vi "RW RxTx.vi"(8 "error in (no error)":errorcluster) -> (0 "error out":errorcluster)   [LabVIEW 2018]
uses:
  RxTx/CCS_RxTx.lvclass
  <vilib>/addons/_JKI Toolkits/Caraya/classes/Assert/Assert Equal Value_Variant.vi
  <vilib>/addons/_JKI Toolkits/Caraya/classes/Test/Test.lvclass
  <vilib>/addons/_JKI Toolkits/Caraya/classes/Assert/Assert.lvclass
panel:
  in  "RxTx in":refnum<class "CCS_RxTx.lvclass">
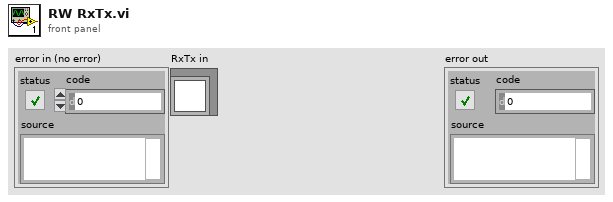
[diagram p1: front panel]
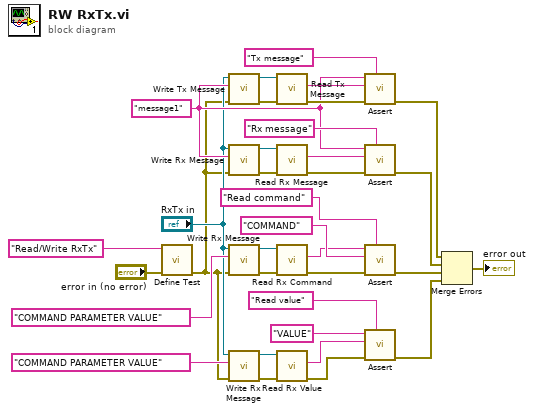
[diagram p0: block diagram]
diagram:
  w19 = "message1" ("Label (VI Title)")
  n1 = call <vilib>:"Define Test.vi"("error in (no error)"="error in (no error)", "Label (VI Title)"="Read/Write RxTx") -> ("error out"=w2:errorcluster)  [unwired: 8 in, 1 out]
  n2 = call "Write Tx Message.vi"("error in (no error)"=w2, "Tx Message"=w19, "RxTx in"="RxTx in") -> ("error out"=w31:errorcluster, "RxTx out"=w23:refnum<class "CCS_RxTx.lvclass">)  [unwired: 7 in]
  n3 = call "Write Rx Message.vi"("error in (no error)"=w2, "Rx Message"=w19, "RxTx in"="RxTx in") -> ("error out"=w28:errorcluster, "RxTx out"=w22:refnum<class "CCS_RxTx.lvclass">)  [unwired: 7 in]
  n4 = call "Write Rx Message.vi"("error in (no error)"=w2, "Rx Message"="COMMAND PARAMETER VALUE" ("Label (VI Title)"), "RxTx in"="RxTx in") -> ("error out"=w16:errorcluster, "RxTx out"=w15:refnum<class "CCS_RxTx.lvclass">)  [unwired: 7 in]
  n5 = call "Write Rx Message.vi"("error in (no error)"=w2, "Rx Message"="COMMAND PARAMETER VALUE" ("Label (VI Title)"), "RxTx in"="RxTx in") -> ("error out"=w9:errorcluster, "RxTx out"=w8:refnum<class "CCS_RxTx.lvclass">)  [unwired: 7 in]
  n6 = call "Read Tx Message.vi"("error in (no error)"=w31, "RxTx in"=w23) -> ("error out"=w30:errorcluster, "Tx Message"=w20:string)  [unwired: 7 in, 1 out]
  n7 = call "Read Rx Message.vi"("error in (no error)"=w28, "RxTx in"=w22) -> ("error out"=w27:errorcluster, "Rx Message"=w21:string)  [unwired: 7 in, 1 out]
  n8 = call "Read Rx Command.vi"("error in (no error)"=w16, "RxTx in"=w15) -> ("error out"=w17:errorcluster, "Rx Command"=w12:string)  [unwired: 7 in, 1 out]
  n9 = call "Read Rx Value.vi"("error in (no error)"=w9, "RxTx in"=w8) -> ("error out"=w1:errorcluster, "Rx value"=w7:string)  [unwired: 7 in, 1 out]
  n10 = call-poly <vilib>:"Assert.vi"("Label"="Tx message" ("Label (VI Title)"), "error in (no error)"=w30, "Y"=w20, "X"=w19) -> ("error out"=w32:errorcluster)  [unwired: 6 in, 1 out]
  n11 = call-poly <vilib>:"Assert.vi"("Label"="Rx message" ("Label (VI Title)"), "error in (no error)"=w27, "Y"=w21, "X"=w19) -> ("error out"=w26:errorcluster)  [unwired: 6 in, 1 out]
  n12 = call-poly <vilib>:"Assert.vi"("Label"="Read command" ("Label (VI Title)"), "error in (no error)"=w17, "Y"="COMMAND" ("Label (VI Title)"), "X"=w12) -> ("error out"=w18:errorcluster)  [unwired: 6 in, 1 out]
  n13 = call-poly <vilib>:"Assert.vi"("Label"="Read value" ("Label (VI Title)"), "error in (no error)"=w1, "Y"=w7, "X"="VALUE" ("Label (VI Title)")) -> ("error out"=w4:errorcluster)  [unwired: 6 in, 1 out]
  n14 = Merge Errors(w32, w26, w18, w4) -> (→"error out":errorcluster)
